vi "Dealt Cards to Card Map.vi"(11 "Dealt Cards":string[](array[string])) -> (2 "Total Hands":i32, 3 "Card Map":i32[][](array[numeric]))   [LabVIEW 2020]
panel:
  # "SUITED"
  # "2"
  # "3"
  # "4"
  # "5"
  # "6"
  # "7"
  # "8"
  # "9"
  # "T"
  # "J"
  # "Q"
  # "K"
  # "A"
  # "A"
  # "K"
  # "Q"
  # "J"
  # "T"
  # "9"
  # "8"
  # "7"
  # "6"
  # "5"
  # "4"
  # "3"
  # "2"
  # "OFFSUIT"
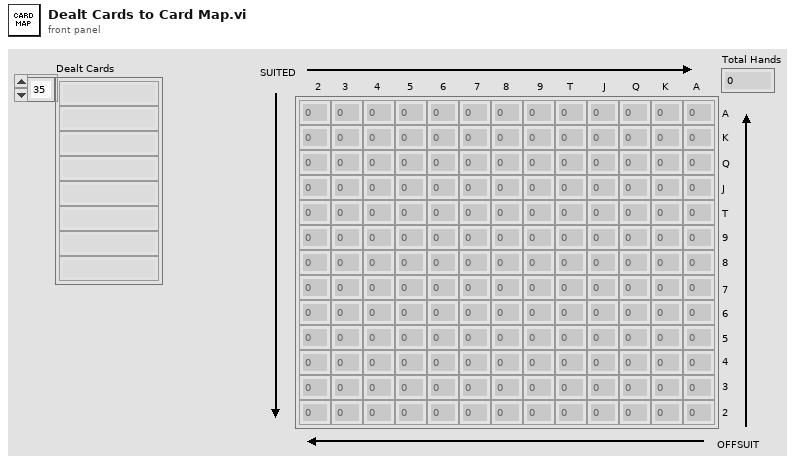
[diagram p1: front panel]
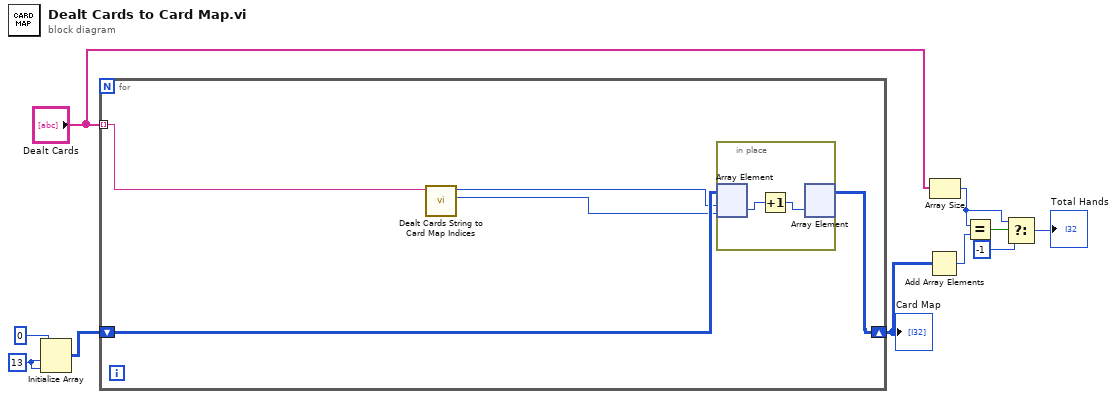
[diagram p0: block diagram]
diagram:
  w10 = 13 ("dimension size")
  n1 = Initialize Array(0, w10, w10) -> (w8:i32[][])
  n2 = for {
    tunnel: "Dealt Cards" -> [w15] mode=indexing
    shift-right: [w12] -> w6
    shift-left: w8 -> [w14]
    n3 = call "Dealt Cards String to Card Map Indices.vi"("Dealt Cards String"=w15) -> ("Index1"=w13:i32, "Index0"=w11:i32)  [unwired: 9 in]
    n4 = in-place {
      n5 = in-place-array #1(w14, w11, w13) -> (w17:i32)
      n6 = Increment(x=w17) -> (x+1=w16:i32)
      n7 = in-place-array #1(w16) -> (w12:i32[][])  [unwired: 2 out]
    }
  }
  "Card Map" <- w6
  n8 = Add Array Elements(numeric array=w6) -> (sum=w5:i32)
  n9 = Array Size(array="Dealt Cards") -> (size(s)=w3:i32)
  n10 = Equal?(x=w3, y=w5) -> (x = y?=w4:bool)
  n11 = Select(t=w3, s=w4, f=-1) -> (s? t:f=→"Total Hands":i32)
